vi "EditConfig.vi"() -> ()   [LabVIEW 2014]
uses:
  <vilib>/Utility/error.llb/DialogType.ctl
  TempConfig.ctl
panel:
  in  "Error In":errorcluster
  in  "Save Button":bool
  in  "Remove Button":bool
  in  "Add Button":bool
  in  "Combo Box":string(combo)
  in  "Cancel Button":bool
  in  "TempConfig":T1
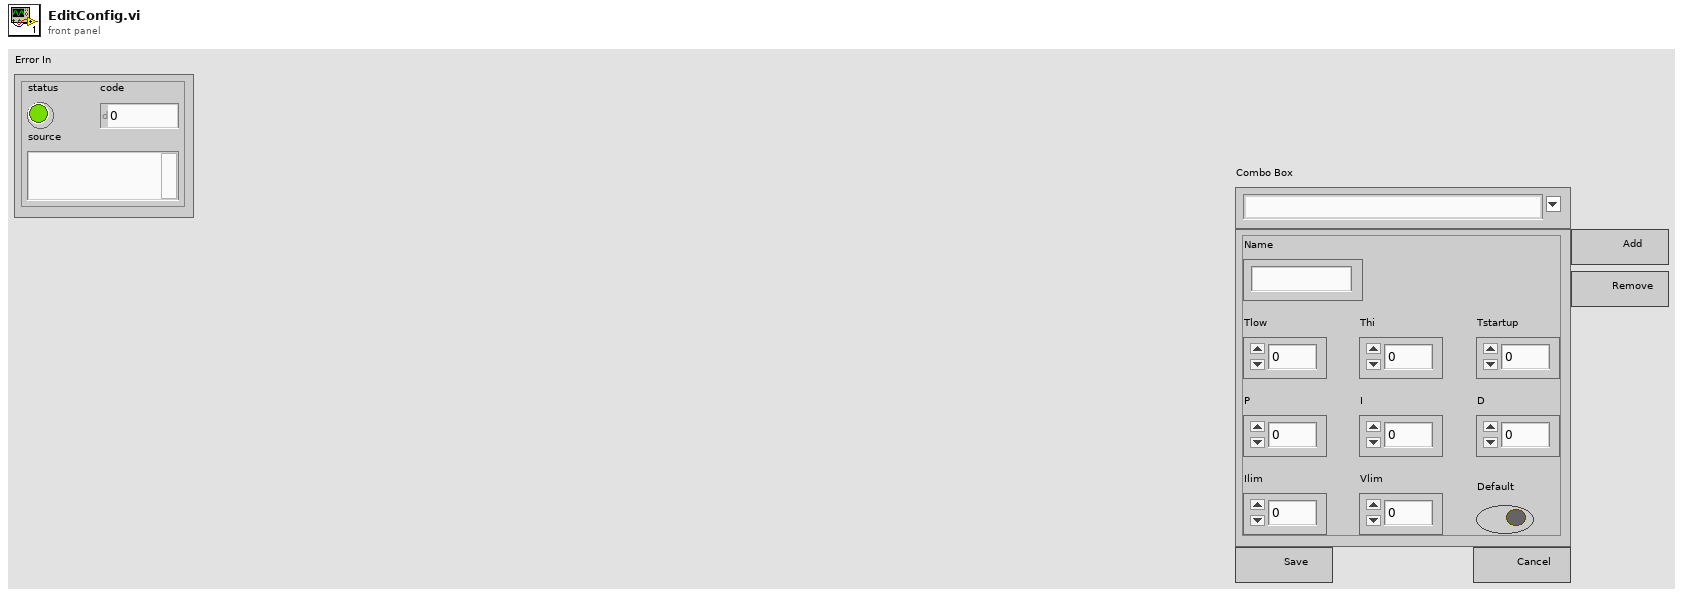
[diagram p1: front panel]
types:
  T1 = typedef "TempConfig.ctl" = cluster{"Name":string, "Thi":dbl, "Tlow":dbl, "Tstartup":dbl, "P":dbl, "I":dbl, "D":dbl, "Ilim":dbl, "Vlim":dbl, "Default":bool}
  T2 = typedef "DialogType.ctl" = u16
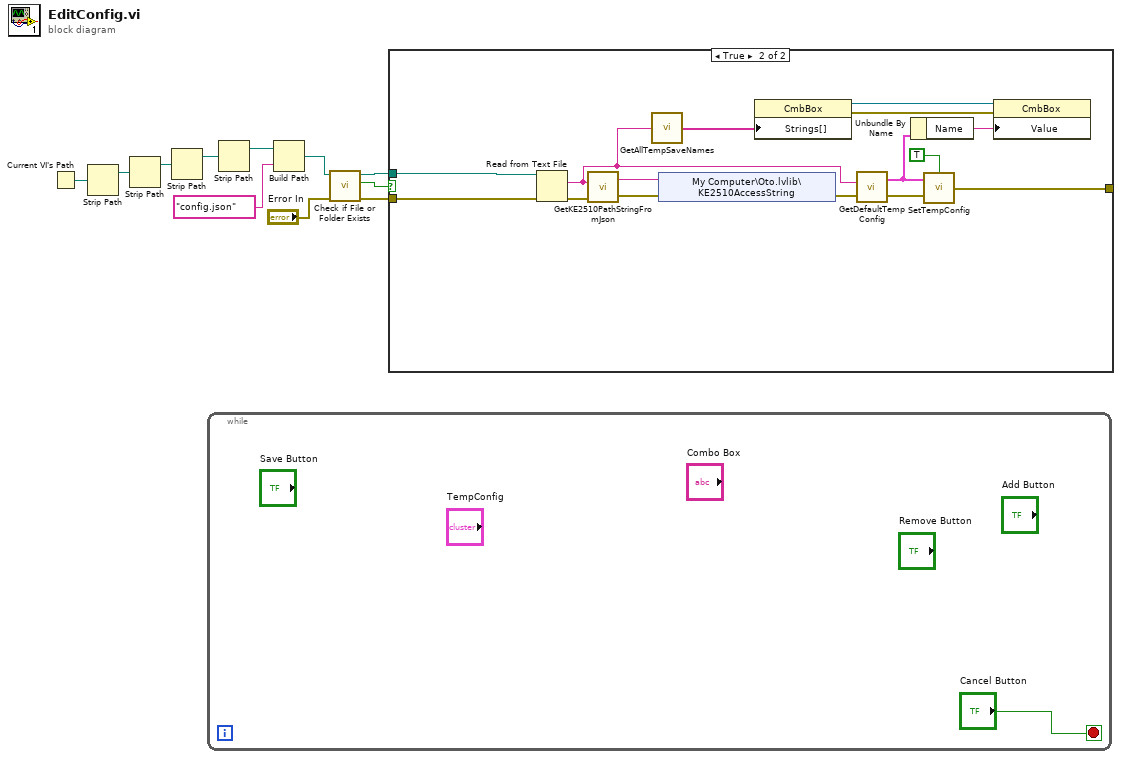
[diagram p0: block diagram]
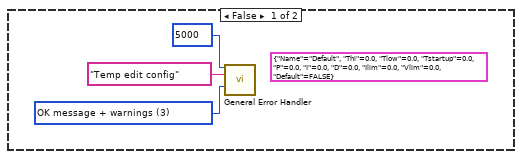
[diagram p2: hidden frame]
diagram:
  n1 = Current VI's Path() -> (path=w11:path)
  n2 = Strip Path(path=w11) -> (stripped path=w2:path)  [unwired: 1 out]
  n3 = Strip Path(path=w2) -> (stripped path=w4:path)  [unwired: 1 out]
  n4 = Strip Path(path=w4) -> (stripped path=w3:path)  [unwired: 1 out]
  n5 = while {
    stop <- "Cancel Button" stop-if-true
  }
  n6 = Strip Path(path=w3) -> (stripped path=w1:path)  [unwired: 1 out]
  n7 = Build Path(base path=w1, name or relative path="config.json") -> (appended path=w5:path)
  n8 = call <vilib>:"Check if File or Folder Exists.vi"("error in (no error)"="Error In", "path"=w5) -> ("error out"=w8:errorcluster, "file or folder exists?"=w9:bool, "dup path"=w10:path)  [unwired: 7 in]
  n9 = case shown="True" w9 {
    tunnel: w10 -> [_ w29]
    tunnel: w8 -> [_ w30]
    tunnel: [_ w27] -> _
    frame False {
      (unwired) T1 {"Name"="Default", "Thi"=0.0, "Tlow"=0.0, "Tstartup"=0.0, "P"=0.0, "I"=0.0, "D"=0.0, "Ilim"=0.0, "Vlim"=0.0, "Default"=FALSE} ("Default configuration")
      w15 = T2 3 items=["no dialog", "OK message", "continue or stop message", "OK message + warnings", "continue/stop + warnings"] ("type of dialog (OK msg:1)")
      n10 = call <vilib>:"General Error Handler.vi"("[error code] (0)"=5000, "[error source] (\" \")"="Temp edit config" ("[error source] (\" \")"), "type of dialog (OK msg:1)"=w15) -> ()  [unwired: 8 in, 5 out]
    }
    frame True {
      n11 = Read from Text File(file (use dialog)=w29, error in=w30) -> (text=w22:string, error out=w26:errorcluster)  [unwired: 2 in, 2 out]
      n12 = call "GetKE2510PathStringFromJson.vi"("Error In"=w26, "JSON"=w22) -> ("Error Out"=w24:errorcluster, "Path String"=w25:string)
      n13 = call "GetAllTempSaveNames.vi"("String"=w22) -> ("Array"=w21:string[])
      n14 = shared-variable "My Computer\\Oto.lvlib\\KE2510AccessString"(w25, error in=w24) -> (error out=w23:errorcluster)
      n15 = property class="CmbBox"("Strings[]"=w21) -> (reference out=w20:refnum<vi>, error out=w19:errorcluster)  [unwired: 2 in]
      n16 = call "GetDefaultTempConfig.vi"("Error In"=w23, "String"=w22) -> ("Error Out"=w28:errorcluster, "TempConfig"=w18:T1)
      n17 = Unbundle By Name(w18) -> ("Name"=w17:string)
      n18 = call "SetTempConfig.vi"("Boolean"=TRUE, "Error In"=w28, "Temp Configuration"=w18) -> ("Error Out"=w27:errorcluster)
      n19 = property class="CmbBox"(reference=w20, error in=w19, "Value"=w17) -> ()  [unwired: 2 out]
    }
  }
